vi "Hitrap_DiagnosticBoxGUI.destructor.vi"(0 "i ref in":refnum<vi>, 5 "error in (no error)":errorcluster) -> (19 "error out":errorcluster)   [LabVIEW 2014, in "Hitrap_DiagnosticBoxGUI.lvlib"]
doc: "This is the destructor of a class.\n\nLicense Agreement for this software:\n\nCopyright (C)\nGesellschaft für Schwerionenforschung, GSI\nPlanckstr. 1\n64291 Darmstadt\nGermany\n\nContact: D.Beck@gsi.de \n\nThis program is free software; you can redistribute it and/or modify it under the terms of the \nGNU General Public License as published by the Free Software Foundation; either version 2 of \nthe license, or (at your option) any later version.\n\nThis program is distributed in the hope that it will be useful, but WITHOUT ANY WARRANTY; \nwithout even the implied warranty of MERCHANTABILITY or FITNESS FOR A PARTICULAR PURPOSE. See the GNU General License for more details (http://www.gnu.org).\n\nGesellschaft für Schwerionenforschung, GSI\nPlanckstr. 1, 64291 Darmstadt, Germany\nFor all questions and ideas contact: M.Richter@gsi.de, H.Brand@gsi.de or D.Beck@gsi.de.\nLast update: 16-JUN-2004"
uses:
  Hitrap_DiagnosticBoxGUI.lvlib
  CS_Core/GUIs/GOGUserGUIs/DeviceBaseGUI/DeviceBaseGUI.lvlib
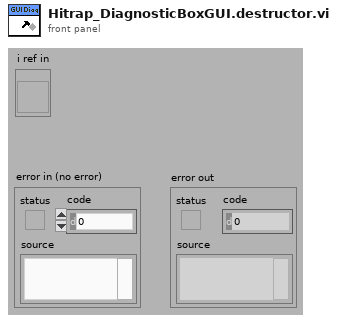
[diagram p1: front panel]
types:
  T1 = enum16{"SetAttribute", "GetAttribute", "CreateAttribute", "DestroyAttribute", "DestroyAllAtributes"}
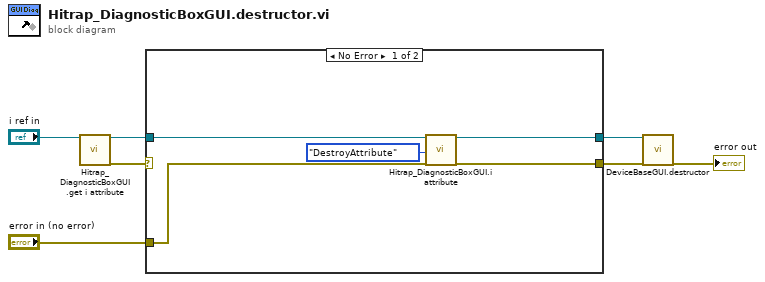
[diagram p0: block diagram]
diagram:
  n1 = call "Hitrap_DiagnosticBoxGUI.get i attribute.vi"("i ref in"="i ref in") -> ("i ref out"=w5:refnum<vi>, "error out"=w4:errorcluster)  [unwired: 16 in, 1 out]
  n2 = case shown="No Error" w4 {
    tunnel: w5 -> [w10 w14]
    tunnel: "error in (no error)" -> [w11 w13]
    tunnel: [w9 w13] -> w3
    tunnel: [w8 w14] -> w1
    frame No Error {
      n3 = call "Hitrap_DiagnosticBoxGUI.i attribute.vi"("VI Refnum"=w10, "Action"=T1."DestroyAttribute", "error in (no error)"=w11) -> ("VI Refnum out"=w8:refnum<vi>, "error out"=w9:errorcluster)  [unwired: 14 in, 1 out]
    }
    frame Error {
    }
  }
  n4 = call "DeviceBaseGUI.destructor.vi"("i ref in"=w1, "error in (no error)"=w3) -> ("error out"=→"error out":errorcluster)  [unwired: 17 in]
